vi "Main.vi"() -> ()   [LabVIEW 2021, in "InstrumentStudio Plug-In Template.lvlib"]
uses:
  InstrumentStudio Plug-In Template.lvlib
  <vilib>/Plug-In SDKs/InstrumentStudio/Plugin Events Enum.ctl
  <vilib>/Plug-In SDKs/InstrumentStudio/Write Edit Time Configuration.vi
  <vilib>/Plug-In SDKs/InstrumentStudio/Write Run Time Configuration.vi
  <vilib>/Plug-In SDKs/InstrumentStudio/Read Edit Time Configuration.vi
  <vilib>/Plug-In SDKs/InstrumentStudio/Read Run Time Configuration.vi
  <vilib>/Plug-In SDKs/InstrumentStudio/Plugin Session.lvclass
  <vilib>/Plug-In SDKs/InstrumentStudio/InstrumentStudio Plugin SDK.lvlib
panel:
  in  "Tab Control":T1(tab)
  in  "Read Selected Sites":bool
  in  "Read Active Pin Map Path":bool
  out "Sites":i32[](array[numeric])
  out "Project Path":path
  in  "Run Write":string
  in  "Write Run Time Config":bool
  in  "Edit Write":string
  in  "Write Edit Time Config":bool
  out "Run Read":string
  in  "Read Run Time Config":bool
  out "Edit Read":string
  in  "Read Edit Time Config":bool
  in  "Read Project Path":bool
  in  "Running":bool
  out "Active Pin Map Path":path
  out "Event Record":i32(listbox)
  in  "Session Id":u64
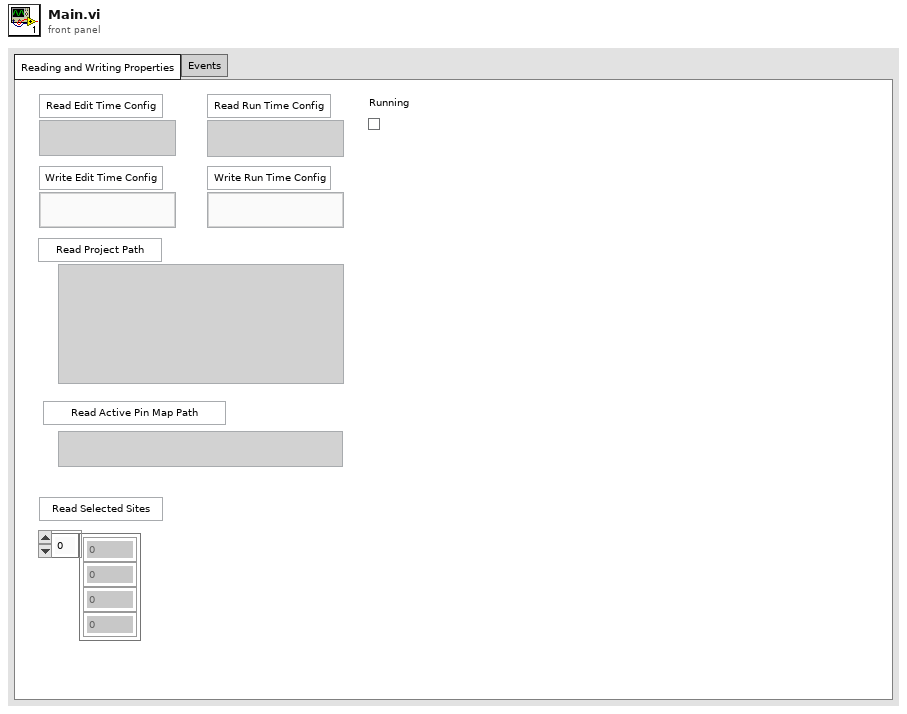
[diagram p1: front panel]
types:
  T1 = enum32{"Reading and Writing Properties", "Events"}
  T2 = typedef "InstrumentStudio Plugin SDK.lvlib/Plugin Events Enum.ctl" = enum32{"Shutdown", "Project Saved", "Stop All Outputs", "Generic Message", "Active Pin Map Changed", "Selected Sites Changed"}
  T3 = typedef "InstrumentStudio Plugin SDK.lvlib/Event Registration Refnum.ctl" = refnum<event-registration>
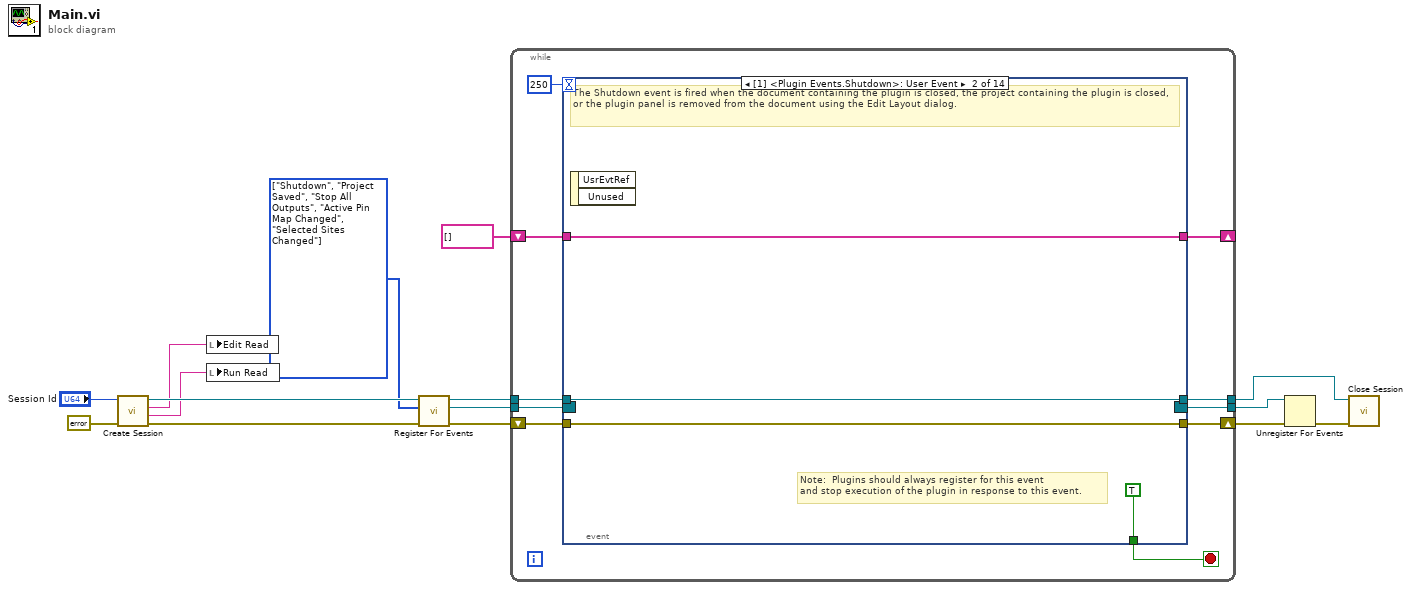
[diagram p0: block diagram]
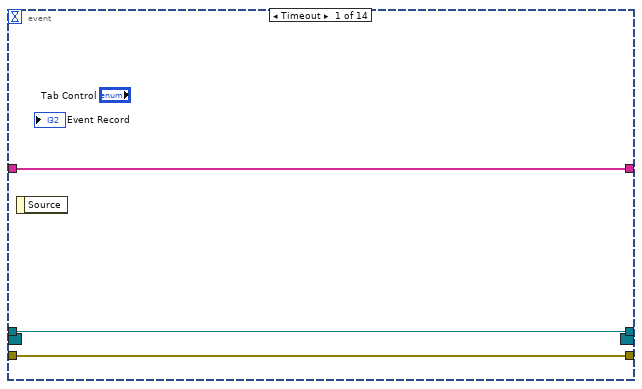
[diagram p2: hidden frame]
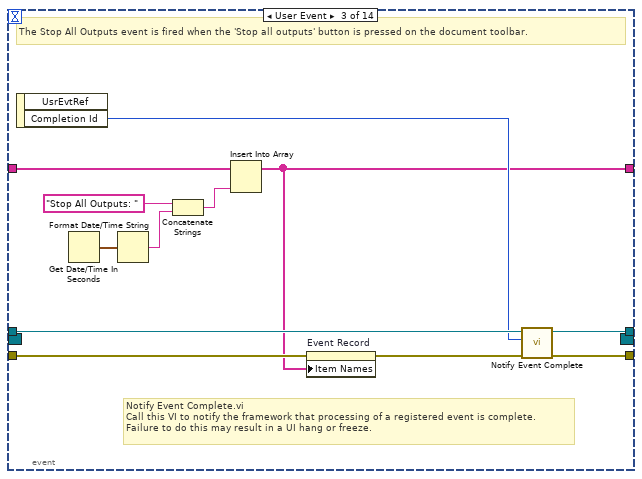
[diagram p3: hidden frame]
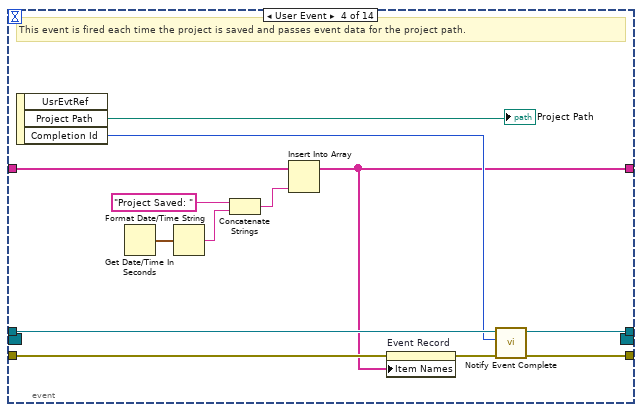
[diagram p4: hidden frame]
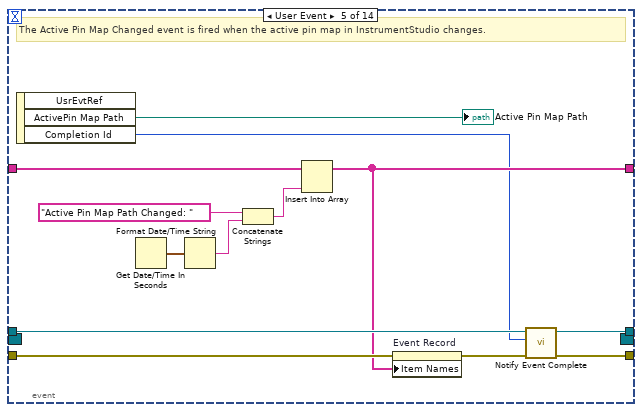
[diagram p5: hidden frame]
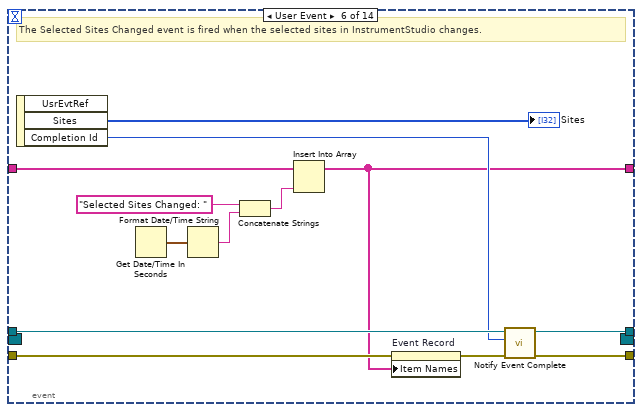
[diagram p6: hidden frame]
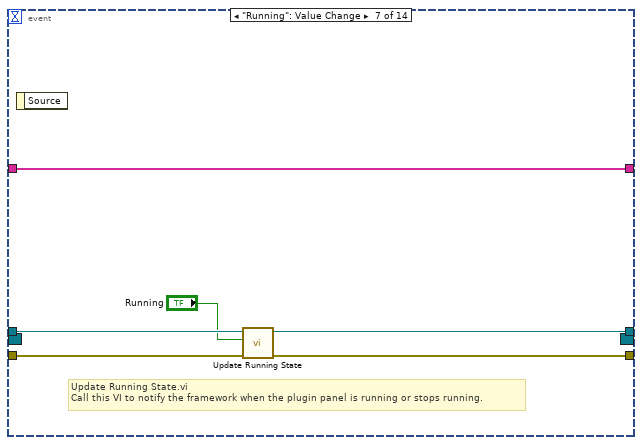
[diagram p7: hidden frame]
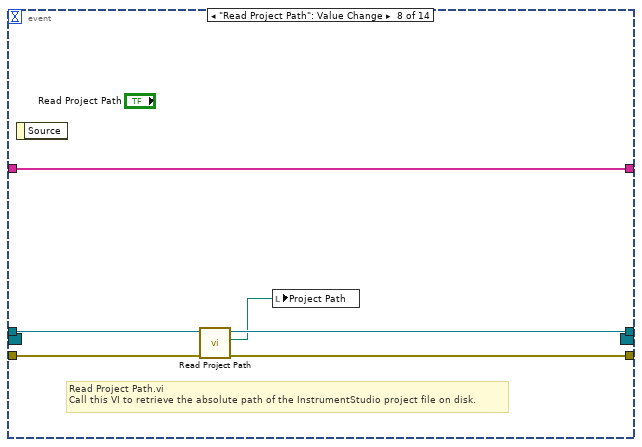
[diagram p8: hidden frame]
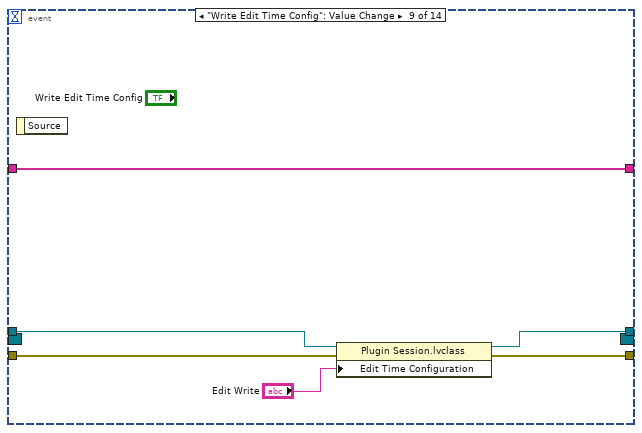
[diagram p9: hidden frame]
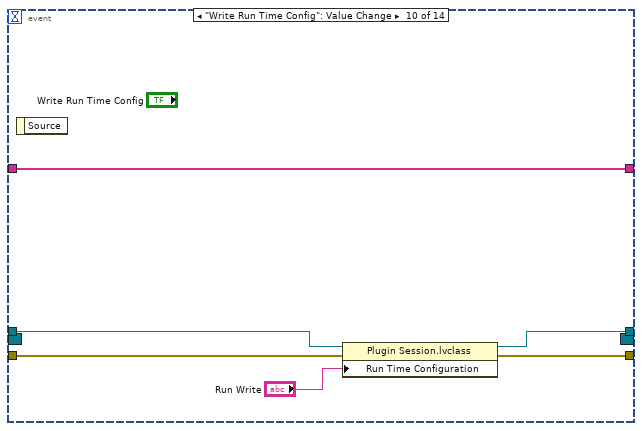
[diagram p10: hidden frame]
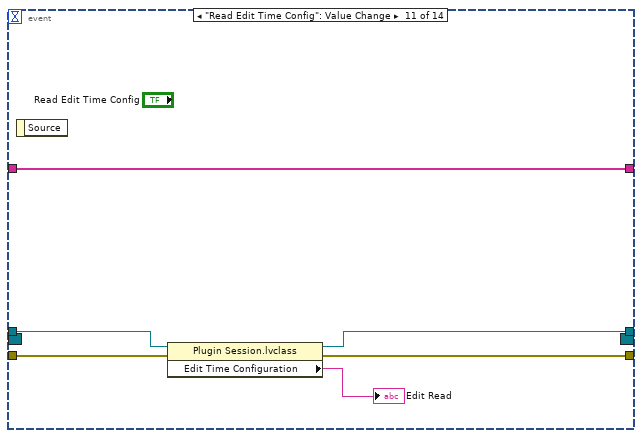
[diagram p11: hidden frame]
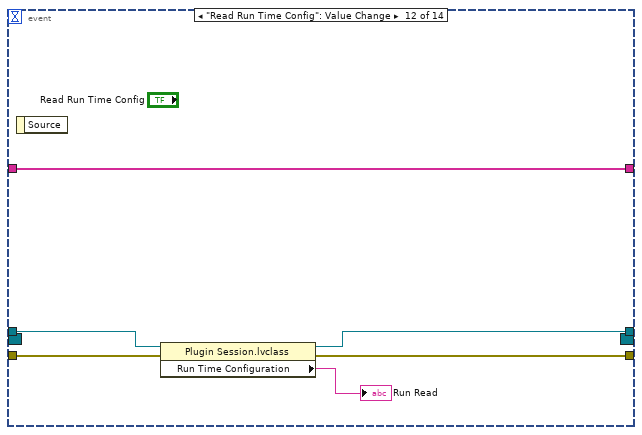
[diagram p12: hidden frame]
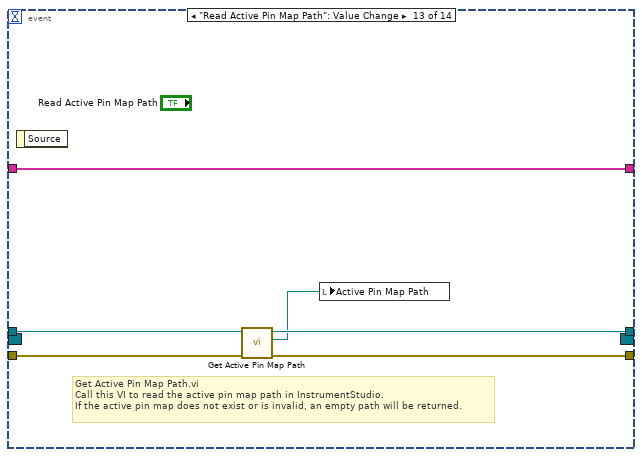
[diagram p13: hidden frame]
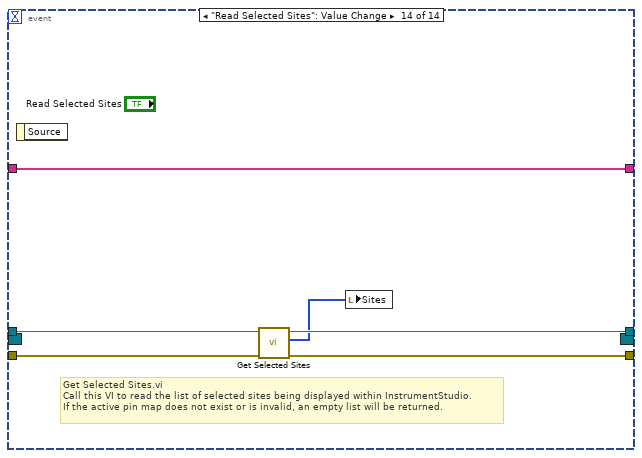
[diagram p14: hidden frame]
diagram:
  w6 = T2[] [enum."Shutdown", enum."Project Saved", enum."Stop All Outputs", enum."Active Pin Map Changed", enum."Selected Sites Changed"] items=["Shutdown", "Project Saved", "Stop All Outputs", "Generic Message", "Active Pin Map Changed", "Selected Sites Changed"] ("Events To Register")
  n1 = call <vilib>:"Create Session.vi"("error in (no error)"=errorcluster {"status"=FALSE, "code"=0, "source"=""}, "Session Id"="Session Id") -> ("error out"=w12:errorcluster, "Run Time Configuration"=w8:string, "Edit Time Configuration"=w7:string, "Session out"=w14:refnum<class "Plugin Session.lvclass">)  [unwired: 5 in, 1 out]
  n2 = local write "Edit Read"(w7) -> ()
  n3 = local write "Run Read"(w8) -> ()
  n4 = call <vilib>:"Register For Events.vi"("error in (no error)"=w12, "Events To Register"=w6, "Session in"=w14) -> ("error out"=w10:errorcluster, "Event Refnum"=w11:T3, "Session out"=w13:refnum<class "Plugin Session.lvclass">)  [unwired: 6 in]
  n5 = while {
    tunnel: w13 -> [w25]
    tunnel: w11 -> [w16]
    shift-right: [w24] -> w3
    shift-left: w10 -> [w21]
    shift-right: [w23] -> _
    shift-left: string[] [] -> [w22]
    tunnel: [w19] -> w4
    tunnel: [w18] -> w5
    stop <- w20 stop-if-true
    n6 = event shown="[1] <Plugin Events.Shutdown>: User Event" {
      selector: w16 -> [_ _ _ _ _ _ _ _ _ _ _ _ _ _]
      dyn-events: [_ _ _ _ _ _ _ _ _ _ _ _ _ _] -> w18
      timeout: 250 -> [_ _ _ _ _ _ _ _ _ _ _ _ _ _]
      tunnel: w25 -> [w28 w32 w44 w57 w70 w82 w89 w95 w97 w104 w110 w116 w124 w130]
      tunnel: [w28 w32 w43 w56 w69 w83 w88 w94 w96 w103 w109 w115 w123 w128] -> w19
      tunnel: [w27 w31 w40 w54 w68 w79 w86 w91 w99 w105 w112 w117 w122 w127] -> w24
      tunnel: [w26 w30 w36 w45 w63 w71 w85 w93 w101 w107 w113 w119 w125 w131] -> w23
      tunnel: w22 -> [w26 w30 w38 w51 w65 w77 w85 w93 w101 w107 w113 w119 w125 w131]
      tunnel: w21 -> [w27 w31 w41 w52 w66 w78 w87 w92 w100 w106 w111 w118 w121 w129]
      tunnel: [_ TRUE _ _ _ _ _ _ _ _ _ _ _ _] -> w20
      event Timeout {
        n7 = event-data() -> ()  [unwired: 1 in, 1 out]
      }
      event User Event {
        # "Note:  Plugins should always register for this event\nand stop execution of the plugin in response to this event."
        # "The Shutdown event is fired when the document containing the plugin is closed, the project containing the plugin is closed, or the plugin panel is removed from the document using the Edit Layout dialog."
        n8 = event-data() -> ()  [unwired: 1 in, 2 out]
      }
      event User Event {
        # "Notify Event Complete.vi\nCall this VI to notify the framework that processing of a registered event is complete. \nFailure to do this may result in a UI hang or freeze."
        # "The Stop All Outputs event is fired when the 'Stop all outputs' button is pressed on the document toolbar."
        n9 = event-data() -> ("Completion Id"=w39:i64)  [unwired: 1 in, 1 out]
        n10 = Get Date/Time In Seconds() -> (seconds since 1Jan1904=w35:timestamp)
        n11 = Format Date/Time String(seconds (now)=w35) -> (date/time string=w34:string)  [unwired: 2 in]
        n12 = Concatenate Strings("Stop All Outputs: ", w34) -> (w37:string)
        n13 = Insert Into Array(array=w38, new element=w37) -> (w36:string[])  [unwired: 1 in]
        n14 = property on="Event Record" class="LstBox (strict)"(error in=w41, "Item Names"=w36) -> (error out=w42:errorcluster)  [unwired: 1 in, 1 out]
        n15 = call <vilib>:"Notify Event Complete.vi"("error in (no error)"=w42, "Completion Id"=w39, "Session in"=w44) -> ("error out"=w40:errorcluster, "Session out"=w43:refnum<class "Plugin Session.lvclass">)  [unwired: 7 in]
      }
      event User Event {
        # "This event is fired each time the project is saved and passes event data for the project path."
        n16 = event-data() -> ("Project Path"=→"Project Path":path, "Completion Id"=w46:i64)  [unwired: 1 in, 1 out]
        n17 = Get Date/Time In Seconds() -> (seconds since 1Jan1904=w50:timestamp)
        n18 = Format Date/Time String(seconds (now)=w50) -> (date/time string=w49:string)  [unwired: 2 in]
        n19 = Concatenate Strings("Project Saved: ", w49) -> (w47:string)
        n20 = Insert Into Array(array=w51, new element=w47) -> (w45:string[])  [unwired: 1 in]
        n21 = property on="Event Record" class="LstBox (strict)"(error in=w52, "Item Names"=w45) -> (error out=w53:errorcluster)  [unwired: 1 in, 1 out]
        n22 = call <vilib>:"Notify Event Complete.vi"("error in (no error)"=w53, "Completion Id"=w46, "Session in"=w57) -> ("error out"=w54:errorcluster, "Session out"=w56:refnum<class "Plugin Session.lvclass">)  [unwired: 7 in]
      }
      event User Event {
        # "The Active Pin Map Changed event is fired when the active pin map in InstrumentStudio changes."
        n23 = event-data() -> ("ActivePin Map Path"=→"Active Pin Map Path":path, "Completion Id"=w58:i64)  [unwired: 1 in, 1 out]
        n24 = Get Date/Time In Seconds() -> (seconds since 1Jan1904=w62:timestamp)
        n25 = Format Date/Time String(seconds (now)=w62) -> (date/time string=w60:string)  [unwired: 2 in]
        n26 = Concatenate Strings("Active Pin Map Path Changed: ", w60) -> (w59:string)
        n27 = Insert Into Array(array=w65, new element=w59) -> (w63:string[])  [unwired: 1 in]
        n28 = property on="Event Record" class="LstBox (strict)"(error in=w66, "Item Names"=w63) -> (error out=w67:errorcluster)  [unwired: 1 in, 1 out]
        n29 = call <vilib>:"Notify Event Complete.vi"("error in (no error)"=w67, "Completion Id"=w58, "Session in"=w70) -> ("error out"=w68:errorcluster, "Session out"=w69:refnum<class "Plugin Session.lvclass">)  [unwired: 7 in]
      }
      event User Event {
        # "The Selected Sites Changed event is fired when the selected sites in InstrumentStudio changes."
        n30 = event-data() -> ("Sites"=→"Sites":i32[], "Completion Id"=w72:i64)  [unwired: 1 in, 1 out]
        n31 = Get Date/Time In Seconds() -> (seconds since 1Jan1904=w74:timestamp)
        n32 = Format Date/Time String(seconds (now)=w74) -> (date/time string=w75:string)  [unwired: 2 in]
        n33 = Concatenate Strings("Selected Sites Changed: ", w75) -> (w76:string)
        n34 = Insert Into Array(array=w77, new element=w76) -> (w71:string[])  [unwired: 1 in]
        n35 = property on="Event Record" class="LstBox (strict)"(error in=w78, "Item Names"=w71) -> (error out=w80:errorcluster)  [unwired: 1 in, 1 out]
        n36 = call <vilib>:"Notify Event Complete.vi"("error in (no error)"=w80, "Completion Id"=w72, "Session in"=w82) -> ("error out"=w79:errorcluster, "Session out"=w83:refnum<class "Plugin Session.lvclass">)  [unwired: 7 in]
      }
      event "Running": Value Change {
        # "Update Running State.vi\nCall this VI to notify the framework when the plugin panel is running or stops running."
        n37 = event-data() -> ()  [unwired: 1 in, 1 out]
        n38 = call <vilib>:"Update Running State.vi"("error in (no error)"=w87, "Is Running"="Running", "Plugin Session in"=w89) -> ("error out"=w86:errorcluster, "Plugin Session out"=w88:refnum<class "Plugin Session.lvclass">)  [unwired: 7 in]
      }
      event "Read Project Path": Value Change {
        # "Read Project Path.vi\nCall this VI to retrieve the absolute path of the InstrumentStudio project file on disk."
        n39 = event-data() -> ()  [unwired: 1 in, 1 out]
        n40 = call <vilib>:"Read Project Path.vi"("error in (no error)"=w92, "Session in"=w95) -> ("error out"=w91:errorcluster, "Project Path"=w90:path, "Session out"=w94:refnum<class "Plugin Session.lvclass">)  [unwired: 7 in]
        n41 = local write "Project Path"(w90) -> ()
      }
      event "Write Edit Time Config": Value Change {
        n42 = event-data() -> ()  [unwired: 1 in, 1 out]
        n43 = property class="Plugin Session.lvclass"(reference=w97, error in=w100, "Edit Time Configuration"="Edit Write") -> (reference out=w96:refnum<class "Plugin Session.lvclass">, error out=w99:errorcluster)
      }
      event "Write Run Time Config": Value Change {
        n44 = event-data() -> ()  [unwired: 1 in, 1 out]
        n45 = property class="Plugin Session.lvclass"(reference=w104, error in=w106, "Run Time Configuration"="Run Write") -> (reference out=w103:refnum<class "Plugin Session.lvclass">, error out=w105:errorcluster)
      }
      event "Read Edit Time Config": Value Change {
        n46 = event-data() -> ()  [unwired: 1 in, 1 out]
        n47 = property class="Plugin Session.lvclass"(reference=w110, error in=w111) -> (reference out=w109:refnum<class "Plugin Session.lvclass">, error out=w112:errorcluster, "Edit Time Configuration"=→"Edit Read":string)
      }
      event "Read Run Time Config": Value Change {
        n48 = event-data() -> ()  [unwired: 1 in, 1 out]
        n49 = property class="Plugin Session.lvclass"(reference=w116, error in=w118) -> (reference out=w115:refnum<class "Plugin Session.lvclass">, error out=w117:errorcluster, "Run Time Configuration"=→"Run Read":string)
      }
      event "Read Active Pin Map Path": Value Change {
        # "Get Active Pin Map Path.vi\nCall this VI to read the active pin map path in InstrumentStudio. \nIf the active pin map does not exist or is invalid, an empty path will be returned."
        n50 = event-data() -> ()  [unwired: 1 in, 1 out]
        n51 = call-dynamic "Get Active Pin Map Path.vi"("error in (no error)"=w121, "Session in"=w124) -> ("error out"=w122:errorcluster, "Active Pin Map Path"=w120:path, "Session out"=w123:refnum<class "Plugin Session.lvclass">)  [unwired: 7 in]
        n52 = local write "Active Pin Map Path"(w120) -> ()
      }
      event "Read Selected Sites": Value Change {
        # "Get Selected Sites.vi\nCall this VI to read the list of selected sites being displayed within InstrumentStudio.\nIf the active pin map does not exist or is invalid, an empty list will be returned."
        n53 = event-data() -> ()  [unwired: 1 in, 1 out]
        n54 = call-dynamic "Get Selected Sites.vi"("error in (no error)"=w129, "Session in"=w130) -> ("error out"=w127:errorcluster, "Selected Sites"=w126:i32[], "Session out"=w128:refnum<class "Plugin Session.lvclass">)  [unwired: 7 in]
        n55 = local write "Sites"(w126) -> ()
      }
    }
  }
  n56 = Unregister For Events(event registration refnum=w5, error in=w3) -> (error out=w2:errorcluster)
  n57 = call <vilib>:"Close Session.vi"("error in (no error)"=w2, "Session in"=w4) -> ()  [unwired: 9 in, 1 out]
